vi "PH_Calorimeter_USB.Get Energy.vi"(0 "i ref in":refnum<vi>, 2 "Raw Data":dbl[][](array[numeric]), 5 "error in (no error)":errorcluster) -> (14 "i ref out":refnum<vi>, 15 "Energy [J]":dbl, 16 "Graph":cluster{dbl[], dbl[]}, 18 "Offset Time [s]":dbl, 19 "error out":errorcluster)   [LabVIEW 2014, in "PH_Calorimeter_USB.lvlib"]
doc: "This VI calculates the result from the Raw data and other information."
uses:
  PH_Calorimeter_USB.lvlib
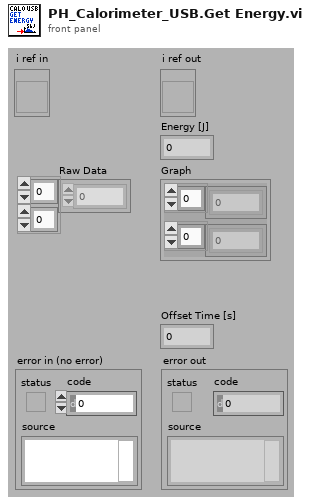
[diagram p1: front panel]
types:
  T1 = typedef "PH_Calorimeter_USB.lvlib/PH_Calorimeter_USB.i attribute.ctl" = cluster{"GUI Refs":cluster{"Delete":refnum<vi>, "Start":refnum<vi>, "Energy":refnum<vi>, "Calorimeter":refnum<vi>, "Trigger":refnum<vi>, "Calo Calibration":refnum<vi>, "Time Base":refnum<vi>, "Device":refnum<vi>, "Graph Raw Data":refnum<vi>, "Graph Result":refnum<vi>}, "DAQ Instance":string, "Data":dbl[][], "Controller Instance":string, "Energy [J]":dbl, "Calorimeter":T2, "Trigger":T3, "Time Base":T4, "Calo Calibration":T5, "Serial Number":string}
  T2 = typedef "PH_Calorimeter_USB.lvlib/PH_Calorimeter_USB.Calorimeter Settings.ctl" = cluster{"Channel":tag, "Min Value [V]":dbl, "Max Value  [V]":dbl}
  T3 = typedef "PH_Calorimeter_USB.lvlib/PH_Calorimeter_USB.Trigger Settings.ctl" = cluster{"Channel":tag, "Min Value [V]":dbl, "Max Value  [V]":dbl, "Level [V]":dbl, "Wait Time [s]":dbl, "Length [Samples]":i32}
  T4 = typedef "PH_Calorimeter_USB.lvlib/PH_Calorimeter_USB.Time Base Settings.ctl" = cluster{"Samples per Channel":i32, "Rate [Hz]":i32}
  T5 = typedef "PH_Calorimeter_USB.lvlib/PH_Calorimeter_USB.Calorimeter Calibration Settings.ctl" = cluster{"T 1/e [s]":dbl, "Sensitivity  [Vs/J]":dbl}
  T6 = cluster{dbl[], "DAQ Data without Offset [V]":dbl[]}
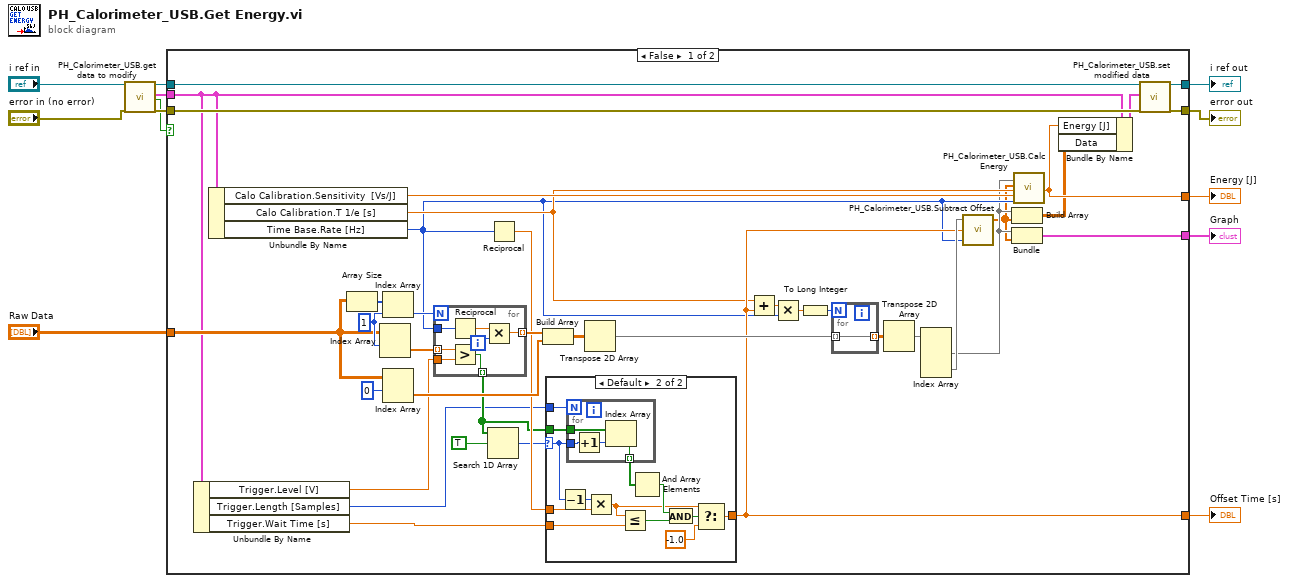
[diagram p0: block diagram]
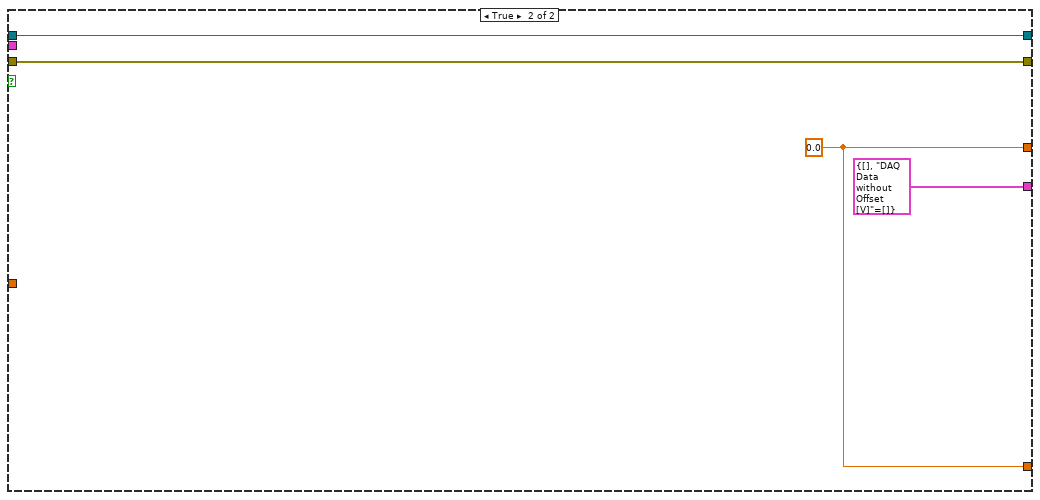
[diagram p3: hidden frame]
diagram:
  n1 = call "PH_Calorimeter_USB.get data to modify.vi"("i ref in"="i ref in", "error in (no error)"="error in (no error)") -> ("i ref out"=w6:refnum<vi>, "i attribute"=w4:T1, "timed out"=w2:bool, "error out"=w8:errorcluster)  [unwired: 14 in]
  n2 = case shown="False" w2 {
    tunnel: [w45 w77] -> w12
    tunnel: [w44 T6 {[], "DAQ Data without Offset [V]"=[]}] -> w11
    tunnel: w8 -> [w26 w79]
    tunnel: [w25 w79] -> w7
    tunnel: w6 -> [w24 w80]
    tunnel: [w23 w80] -> w5
    tunnel: w4 -> [w13 _]
    tunnel: [w21 w77] -> w3
    tunnel: "Raw Data" -> [w17 _]
    frame False {
      w35 = 1 ("index")
      n3 = Unbundle By Name(w13) -> ("Trigger.Level [V]"=w14:dbl, "Trigger.Length [Samples]"=w15:i32, "Trigger.Wait Time [s]"=w16:dbl)
      n4 = Unbundle By Name(w13) -> ("Calo Calibration.Sensitivity  [Vs/J]"=w29:dbl, "Calo Calibration.T 1/e [s]"=w28:dbl, "Time Base.Rate [Hz]"=w27:i32)
      n5 = Array Size(array=w17) -> (size(s)=w30:i32[])
      n6 = Index Array(array=w17, index (row)=w35) -> (element=w33:dbl[])  [unwired: 1 in]
      n7 = Index Array(array=w30, index=w35) -> (element=w31:i32)
      n8 = Index Array(array=w17, index (row)=0) -> (element=w43:dbl[])  [unwired: 1 in]
      n9 = for {
        N: w31 -> [_]
        tunnel: [w75] -> w42 mode=indexing
        tunnel: w27 -> [w73]
        tunnel: w33 -> [w72] mode=indexing
        tunnel: w14 -> [w71]
        tunnel: [w70] -> w36 mode=indexing
        i -> [w76]
        n10 = Reciprocal(x=w73) -> (1/x=w74:dbl)
        n11 = Greater?(x=w72, y=w71) -> (0:w70:bool)
        n12 = Multiply(x=w74, y=w76) -> (x*y=w75:dbl)
      }
      n13 = Search 1D Array(1D array=w36, element=TRUE) -> (index of element=w37:i32)  [unwired: 1 in]
      n14 = Reciprocal(x=w27) -> (1/x=w38:dbl)
      n15 = Build Array(w42, w43) -> (w46:dbl[][])
      n16 = case shown="Default" w37 {
        selector: w37 -> [w51 w60]
        tunnel: w36 -> [_ w64]
        tunnel: w38 -> [_ w62]
        tunnel: [w51 w54] -> w45
        tunnel: w16 -> [_ w59]
        tunnel: w15 -> [_ w52]
        frame -1 {
        }
        frame Default {
          n17 = Decrement(x=w60) -> (x-1=w61:i32)
          n18 = for {
            N: w52 -> [_]
            tunnel: w64 -> [w68]
            tunnel: w60 -> [w67]
            tunnel: [w65] -> w63 mode=indexing
            n19 = Increment(x=w67) -> (x+1=w66:i32)
            n20 = Index Array(array=w68, index=w66) -> (element=w65:bool)
          }
          n21 = Multiply(x=w61, y=w62) -> (x*y=w55:dbl)
          n22 = Less Or Equal?(x=w55, y=w59) -> (x <= y?=w58:bool)
          n23 = And Array Elements(Boolean array=w63) -> (logical AND=w57:bool)
          n24 = And(x=w57, y=w58) -> (x .and. y?=w56:bool)
          n25 = Select(t=w55, s=w56, f=-1.0) -> (s? t:f=w54:dbl)
        }
      }
      n26 = Transpose 2D Array(2D array=w46) -> (transposed array=w47:dbl[][])
      n27 = Add(x=w28, y=w45) -> (x+y=w39:dbl)
      n28 = Multiply(x=w39, y=w27) -> (x*y=w40:dbl)
      n29 = To Long Integer(number=w40) -> (32bit integer=w41:i32)
      n30 = for {
        N: w41 -> [_]
        tunnel: w47 -> [w69] mode=indexing
        tunnel: [w69] -> w49 mode=indexing
      }
      n31 = Transpose 2D Array(2D array=w49) -> (transposed array=w48:dbl[][])
      n32 = Index Array(array=w48) -> (element #1=w20:dbl[], element #2=w50:dbl[])  [unwired: 4 in]
      n33 = call "PH_Calorimeter_USB.Subtract Offset.vi"("Rate [Hz]"=w27, "Offset time [s]"=w45, "DAQ Data [V]"=w50) -> ("DAQ Data without Offset [V]"=w19:dbl[])  [unwired: 1 in, 1 out]
      n34 = Build Array(w20, w19) -> (w18:dbl[][])
      n35 = Bundle(w20, "DAQ Data without Offset [V]"=w19) -> (w44:T6)  [unwired: 1 in]
      n36 = call "PH_Calorimeter_USB.Calc Energy.vi"("Time scale [s]"=w20, "Data without Offset"=w19, "T 1/E [s]"=w28, "sensitivity"=w29, "Output Rate [Hz]"=w27) -> ("Energy [J]"=w21:dbl)  [unwired: 14 in]
      n37 = Bundle By Name(cluster=w13, "Energy [J]"=w21, "Data"=w18) -> (w22:T1)
      n38 = call "PH_Calorimeter_USB.set modified data.vi"("i ref in"=w24, "i attribute"=w22, "error in (no error)"=w26) -> ("i ref out"=w23:refnum<vi>, "error out"=w25:errorcluster)  [unwired: 15 in]
    }
    frame True {
      w77 = 0.0 ("Energy [J]")
    }
  }
  "Offset Time [s]" <- w12
  "Graph" <- w11
  "Energy [J]" <- w3
  "i ref out" <- w5
  "error out" <- w7
